vi "split_string.vi"(11 "String":string) -> (0 "Splitted string tokens":T2, 3 "Splitted string":T1)   [LabVIEW 2021]
uses:
  Controls/SplittedStringTokens.ctl
  Controls/Classes.ctl
  Controls/SplittedString.ctl
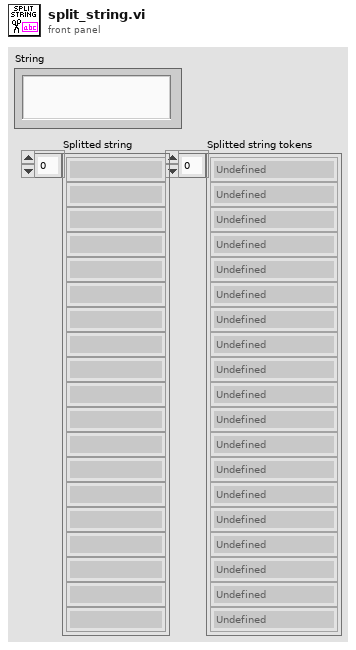
[diagram p1: front panel]
types:
  T1 = typedef "SplittedString.ctl" = string[]
  T2 = typedef "SplittedStringTokens.ctl" = T3[]
  T3 = typedef "Classes.ctl" = enum16{"Undefined", "Left paren", "Right paren", "Number", "Operator", "High level function", "Variable", "End of expression"}
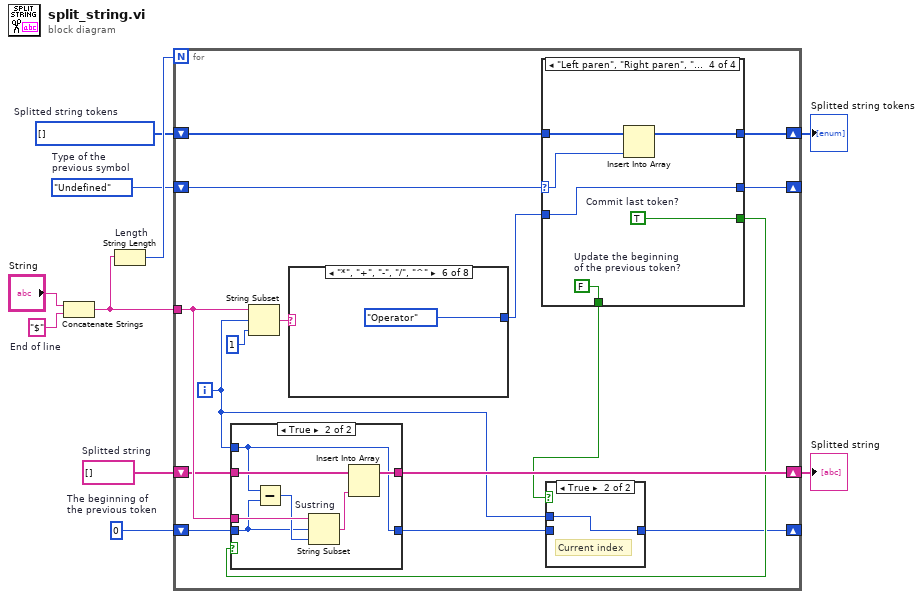
[diagram p0: block diagram]
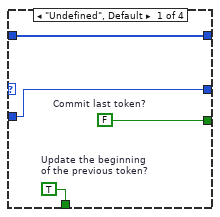
[diagram p3: hidden frame]
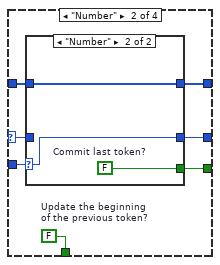
[diagram p4: hidden frame]
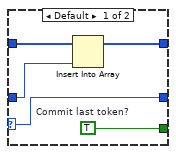
[diagram p5: hidden frame]
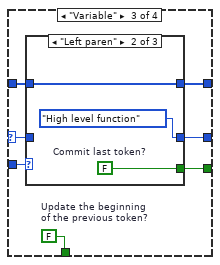
[diagram p6: hidden frame]
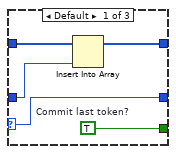
[diagram p7: hidden frame]
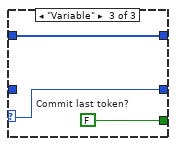
[diagram p8: hidden frame]
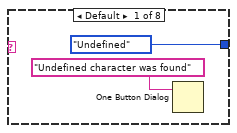
[diagram p10: hidden frame]
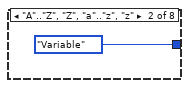
[diagram p11: hidden frame]
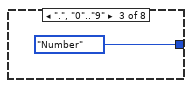
[diagram p12: hidden frame]
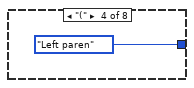
[diagram p13: hidden frame]
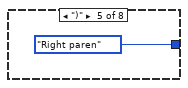
[diagram p14: hidden frame]
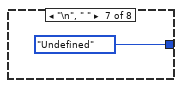
[diagram p15: hidden frame]
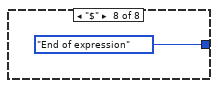
[diagram p16: hidden frame]
diagram:
  w3 = "$"  # End of line
  w6 = T2 [] items=["Undefined", "Left paren", "Right paren", "Number", "Operator", "High level function", "Variable", "End of expression"]  # Splitted string tokens
  w7 = T1 []  # Splitted string
  w8 = Classes."Undefined"  # Type of the  previous symbol
  w9 = 0  # The beginning of  the previous token
  n1 = Concatenate Strings("String", w3) -> (w1:string)
  n2 = String Length "Length"(string=w1) -> (length=w10:i32)
  n3 = for {
    N: w10 -> [_]
    tunnel: w1 -> [w23]
    shift-right: [w13] -> _
    shift-left: w9 -> [w24]
    shift-right: [w17] -> _
    shift-left: w8 -> [w20]
    shift-right: [w21] -> w4
    shift-left: w7 -> [w22]
    shift-right: [w15] -> w5
    shift-left: w6 -> [w16]
    i -> [w11]
    n4 = String Subset(string=w23, offset (0)=w11, length (rest)=1 ("length (rest)")) -> (substring=w25:string)
    n5 = case shown="\"*\", \"+\", \"-\", \"/\", \"^\"" w25 {
      tunnel: [Classes."Undefined" ("Enum") Classes."Variable" ("Enum") Classes."Number" ("Enum") Classes."Left paren" ("Enum") Classes."Right paren" ("Enum") Classes."Operator" ("Enum") Classes."Undefined" ("Enum") Classes."End of expression" ("Enum")] -> w19
      frame Default {
        n6 = One Button Dialog(message="Undefined character was found") -> ()  [unwired: 1 in, 1 out]
      }
      frame "A".."Z", "Z", "a".."z", "z" {
      }
      frame ".", "0".."9" {
      }
      frame "(" {
      }
      frame ")" {
      }
      frame "*", "+", "-", "/", "^" {
      }
      frame "\n", " " {
      }
      frame "$" {
      }
    }
    n7 = case shown="\"Left paren\", \"Right paren\", \"Operator\", \"High level function\", \"End of expression\"" w20 {
      selector: w20 -> [_ w35 w50 w67]
      tunnel: w19 -> [w31 w39 w54 w68]
      tunnel: [w30 w34 w49 w71] -> w18
      tunnel: [w31 w38 w53 w68] -> w17
      tunnel: w16 -> [w32 w37 w52 w70]
      tunnel: [w32 w36 w51 w69] -> w15
      tunnel: [w29 w33 w48 w66] -> w12
      frame "Undefined", Default {
        w29 = TRUE  # Update the beginning  of the previous token?
        w30 = FALSE  # Commit last token?
      }
      frame "Number" {
        w33 = FALSE  # Update the beginning  of the previous token?
        n8 = case shown="\"Number\"" w39 {
          selector: w39 -> [w41 w46]
          tunnel: [w44 w47] -> w34
          tunnel: [w41 w46] -> w38
          tunnel: w37 -> [w43 w45]
          tunnel: [w42 w45] -> w36
          tunnel: w35 -> [w40 _]
          frame Default {
            w44 = TRUE  # Commit last token?
            n9 = Insert Into Array(array=w43, new element=w40) -> (w42:T2)  [unwired: 1 in]
          }
          frame "Number" {
            w47 = FALSE  # Commit last token?
          }
        }
      }
      frame "Variable" {
        w48 = FALSE  # Update the beginning  of the previous token?
        n10 = case shown="\"Left paren\"" w54 {
          selector: w54 -> [w56 _ w63]
          tunnel: [w59 w62 w65] -> w49
          tunnel: [w56 Classes."High level function" ("Enum") w63] -> w53
          tunnel: w52 -> [w58 w61 w64]
          tunnel: [w57 w61 w64] -> w51
          tunnel: w50 -> [w55 _ _]
          frame Default {
            w59 = TRUE  # Commit last token?
            n11 = Insert Into Array(array=w58, new element=w55) -> (w57:T2)  [unwired: 1 in]
          }
          frame "Left paren" {
            w62 = FALSE  # Commit last token?
          }
          frame "Variable" {
            w65 = FALSE  # Commit last token?
          }
        }
      }
      frame "Left paren", "Right paren", "Operator", "High level function", "End of expression" {
        w66 = FALSE  # Update the beginning  of the previous token?
        w71 = TRUE  # Commit last token?
        n12 = Insert Into Array(array=w70, new element=w67) -> (w69:T2)  [unwired: 1 in]
      }
    }
    n13 = case shown="True" w18 {
      tunnel: [w73 w74] -> w14
      tunnel: w24 -> [w73 w75]
      tunnel: w11 -> [_ w74]
      tunnel: w23 -> [_ w80]
      tunnel: w22 -> [w72 w77]
      tunnel: [w72 w78] -> w21
      frame False {
      }
      frame True {
        n14 = Subtract(x=w74, y=w75) -> (x-y=w79:i32)
        n15 = String Subset "Sustring"(string=w80, offset (0)=w75, length (rest)=w79) -> (substring=w76:string)
        n16 = Insert Into Array "Insert Into Array"(array=w77, new element=w76) -> (w78:T1)  [unwired: 1 in]
      }
    }
    n17 = case shown="True" w12 {
      tunnel: w14 -> [w27 _]
      tunnel: [w27 w28] -> w13
      tunnel: w11 -> [_ w28]
      frame False {
        # "Old index"
      }
      frame True {
        # "Current index"
      }
    }
  }
  "Splitted string tokens" <- w5
  "Splitted string" <- w4
